vi "Errorbar2000.vi"   [LabVIEW 2013]
uses:
  <vilib>/Heliosphere Research LLC/Advanced Plotting Toolkit/Advanced Plotting Toolkit.lvlib
types:
  T1 = typedef "Advanced Plotting Toolkit.lvlib/PlotID.ctl" = i32
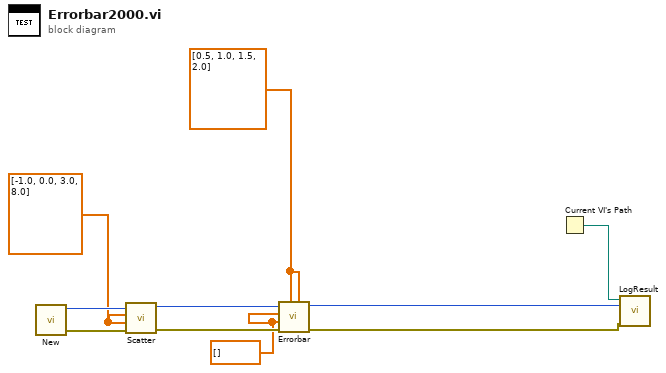
[diagram p0: block diagram]
diagram:
  w1 = dbl[] [] ("Y Data")
  w2 = dbl[] [0.5, 1.0, 1.5, 2.0] ("X Errors")
  w3 = dbl[] [-1.0, 0.0, 3.0, 8.0] ("X Data")
  n1 = call <vilib>:"New.vi"() -> ("error out"=w4:errorcluster, "Plot ID"=w7:T1)  [unwired: 10 in]
  n2 = call <vilib>:"Scatter.vi"("error in (no error)"=w4, "Y Data"=w3, "X Data"=w3, "Plot ID"=w7) -> ("error out"=w5:errorcluster, "Plot ID Out"=w6:T1)  [unwired: 6 in]
  n3 = call <vilib>:"Errorbar.vi"("Y Errors"=w2, "X Errors"=w2, "error in (no error)"=w5, "Y Data"=w1, "X Data"=w1, "Plot ID"=w6) -> ("error out"=w8:errorcluster, "Plot ID out"=w9:T1)  [unwired: 4 in]
  n4 = Current VI's Path() -> (path=w10:path)
  n5 = call "LogResult.vi"("Test Result"=w8, "Test Artifact"=w9, "VI Path"=w10) -> ()  [unwired: 9 in]
